vi "Maj Matrix.vi"(10 "Pixel :":u8[](array[numeric]), 11 "Palette :":T1(array[cluster])) -> (1 "Matrix":u8[](array[numeric]))   [LabVIEW 2014]
panel:
  out "Oct Mx P1 2":u8
  out "Oct Mx P1":u8
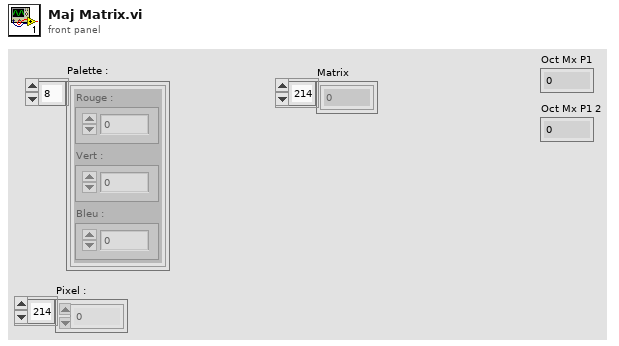
[diagram p1: front panel]
types:
  T1 = cluster{"Rouge : ":u8, "Vert :":u8, "Bleu :":u8}[]
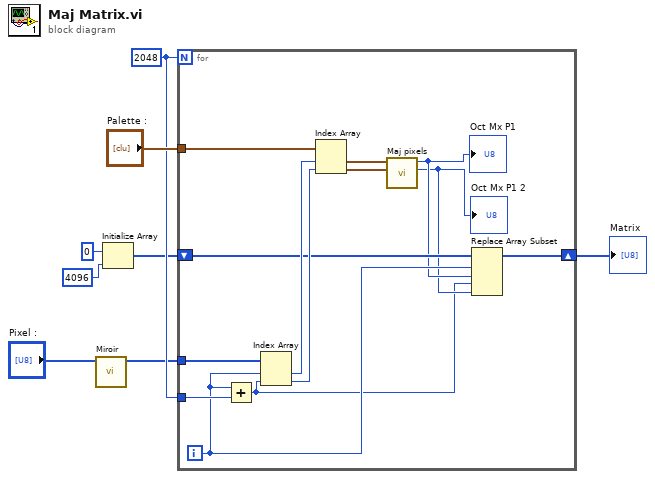
[diagram p0: block diagram]
diagram:
  w7 = 2048
  n1 = call "Miroir.vi"("Pixel"="Pixel :") -> ("Pixel Miroir"=w1:u8[])  [unwired: 10 in]
  n2 = Initialize Array(u8 0, 4096) -> (w4:u8[])
  n3 = for {
    N: w7 -> [_]
    tunnel: "Palette :" -> [w19]
    tunnel: w1 -> [w21]
    tunnel: w7 -> [w20]
    shift-right: [w13] -> w3
    shift-left: w4 -> [w14]
    i -> [w12]
    n4 = Add(x=w12, y=w20) -> (x+y=w9:i32)
    n5 = Index Array(array=w21, index #1=w12, index #2=w9) -> (element #1=w18:u8, element #2=w17:u8)
    n6 = Index Array(array=w19, index #1=w18, index #2=w17) -> (element #1=w16:cluster{"Rouge : ":u8, "Vert :":u8, "Bleu :":u8}, element #2=w15:cluster{"Rouge : ":u8, "Vert :":u8, "Bleu :":u8})
    n7 = call "Maj pixels.vi"("Pixel  B"=w15, "Pixel H"=w16) -> ("Oct Mx P1 2"=w10:u8, "Oct Mx P1"=w11:u8)  [unwired: 8 in]
    "Oct Mx P1" <- w11
    "Oct Mx P1 2" <- w10
    n8 = Replace Array Subset(array=w14, new element #1=w11, index #1=w12, new element #2=w10, index #2=w9) -> (w13:u8[])
  }
  "Matrix" <- w3
